vi "test26-MappingRelationshipByLocalRegistration_WithSubcriberName.vi"(8 "error in (no error)":errorcluster, 11 "TestCase in":refnum<class "testcase-CSMBroadcast.lvclass">) -> (0 "error out":errorcluster, 3 "TestCase out":refnum<class "testcase-CSMBroadcast.lvclass">)   [LabVIEW 2017, in "testcase-CSMBroadcast.lvclass"]
uses:
  testcase-CSMBroadcast.lvclass
  caa41fc0-4920-4570-a7eb-0567c3b7bd6c.vi
  <vilib>/addons/_JKI Toolkits/VI Tester/TestCase.llb/TestCase.lvclass
  src/user.lib/_NEVSTOP/Communicable State Machine(CSM)/Communicable State Machine.lvlib
  CSM/CSM-Testcase.lvlib
  C:/Program Files (x86)/National Instruments/LabVIEW 2017/vi.lib/addons/_JKI Toolkits/VI Tester/TestCase.llb/TestCase.lvclass
panel:
  out "Loop Count":i32
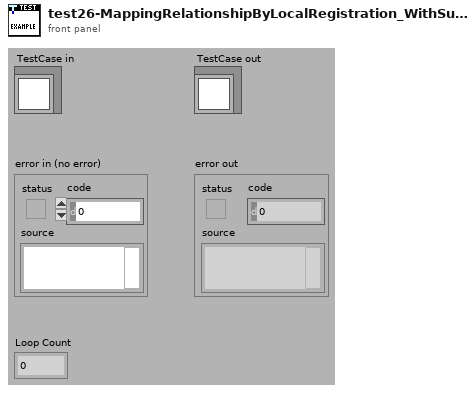
[diagram p1: front panel]
types:
  T1 = cluster{"Status":string, "Source CSM":string, "Target CSM":string, "Target API":string}[]
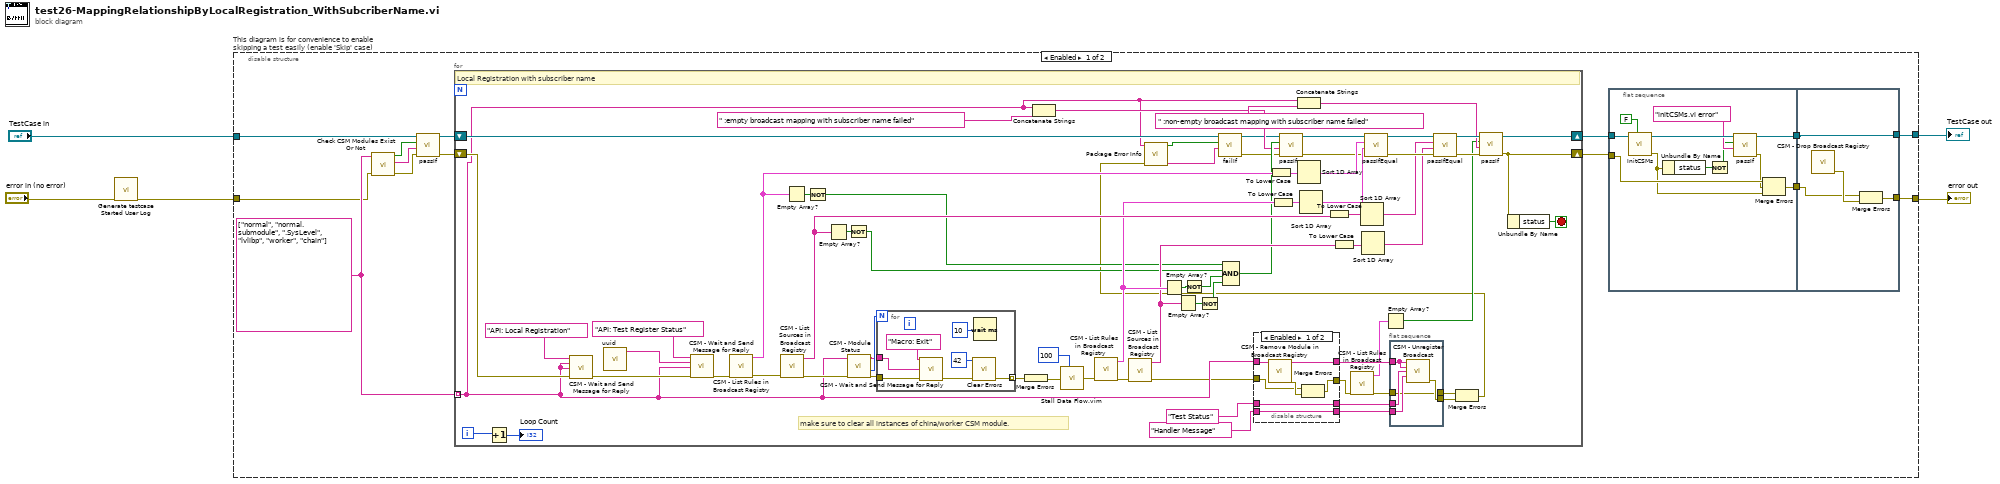
[diagram p0: block diagram]
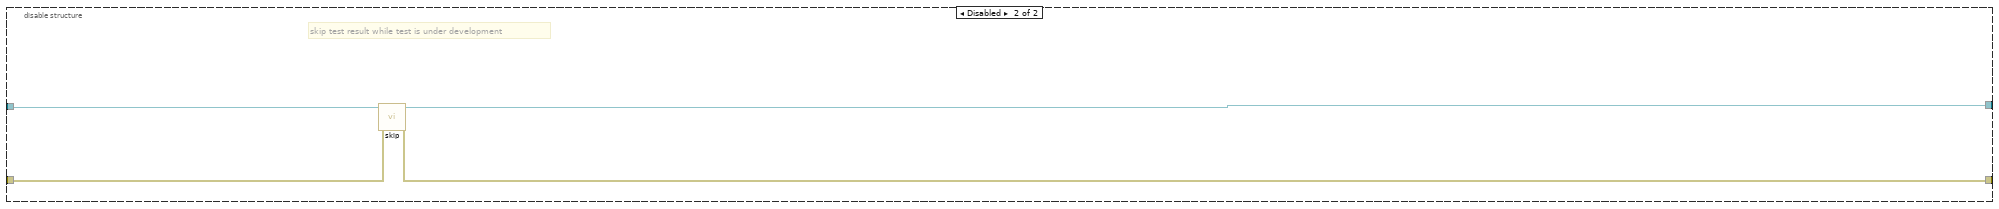
[diagram p3: hidden frame]
diagram:
  n1 = call "Generate testcase Started User Log.vi"("Error In"="error in (no error)") -> ("error out"=w1:errorcluster)  [unwired: 10 in]
  n2 = disable-structure "This diagram is for convenience to enable skipping a test easily (enable 'Skip' case)" shown="Enabled" {
    disable-tunnel: "TestCase in" -> [w15 w132]
    disable-tunnel: [w7 w130] -> w2
    disable-tunnel: [w6 w131] -> w4
    disable-tunnel: w1 -> [w13 w129]
    frame Enabled {
      w16 = string[] ["normal", "normal.submodule", ".SysLevel", "lvlibp", "worker", "chain"]
      n3 = call "Check CSM Modules Exist Or Not.vi"("error in"=w13, "CSM names in"=w16) -> ("error out"=w17:errorcluster, "Debug string"=w18:string, "All Modules Exist?"=w19:bool)  [unwired: 7 in]
      n4 = call-dynamic "passIf.vi"("error in (no error)"=w17, "message (\"\")"=w18, "pass"=w19, "TestCase in"=w15) -> ("error out"=w12:errorcluster, "TestCase out"=w14:refnum<class "testcase-CSMBroadcast.lvclass">)  [unwired: 6 in]
      n5 = for {
        tunnel: w16 -> [w41] mode=indexing
        shift-right: [w71] -> w9
        shift-left: w14 -> [w52]
        shift-right: [w72] -> w8
        shift-left: w12 -> [w62]
        i -> [w86]
        stop <- w99 stop-if-true
        # "make sure to clear all instances of china/worker CSM module."
        # "Local Registration with subscriber name"
        n6 = Increment(x=w86) -> (x+1=→"Loop Count":i32)
        n7 = call "CSM - Wait and Send Message for Reply.vi"("State"="API: Local Registration", "Arguments (\"\")"=w41, "Target Module"=w41, "Error In (No Error)"=w62) -> ("error out"=w104:errorcluster)  [unwired: 8 in, 3 out]
        n8 = call "uuid.vi"() -> ("UUID"=w102:string)  [unwired: 11 in]
        n9 = call "CSM - Wait and Send Message for Reply.vi"("State"="API: Test Register Status", "Arguments (\"\")"=w102, "Target Module"=w41, "Error In (No Error)"=w104) -> ("error out"=w101:errorcluster)  [unwired: 8 in, 3 out]
        n10 = call "CSM - List Rules in Broadcast Registry.vi"("error in (no error)"=w101) -> ("error out"=w98:errorcluster, "Rule Entries"=w84:T1)  [unwired: 8 in, 1 out]
        n11 = call "CSM - List Sources in Broadcast Registry.vi"("error in (no error)"=w98) -> ("error out"=w67:errorcluster, "Broadcast Names"=w81:string[])  [unwired: 9 in]
        n12 = Empty Array?(array=w84) -> (empty?=w83:bool)
        n13 = Not(x=w83) -> (.not. x?=w76:bool)
        n14 = Empty Array?(array=w81) -> (empty?=w82:bool)
        n15 = Not(x=w82) -> (.not. x?=w75:bool)
        n16 = call "CSM - Module Status.vi"("Error In"=w67, "CSM Name"=w41) -> ("error out"=w68:errorcluster, "#Nodes"=w70:i32, "CSM Name (Dup)"=w69:string)  [unwired: 5 in, 2 out]
        n17 = for {
          N: w70 -> [_]
          tunnel: w69 -> [w127]
          tunnel: w68 -> [w126]
          tunnel: [w124] -> w100 mode=indexing
          n18 = call "CSM - Wait and Send Message for Reply.vi"("State"="Macro: Exit", "Target Module"=w127, "Error In (No Error)"=w126) -> ("error out"=w125:errorcluster)  [unwired: 9 in, 3 out]
          n19 = call <vilib>:"Clear Errors.vi"("error in (no error)"=w125, "specific error code to clear (0: all)"=42) -> ("error out"=w124:errorcluster)  [unwired: 4 in, 1 out]
          n20 = Wait (ms)(milliseconds to wait=u32 10) -> ()  [unwired: 1 out]
        }
        n21 = Merge Errors(w100) -> (w56:errorcluster)
        n22 = Concatenate Strings(w41, " :empty broadcast mapping with subscriber name failed" ("string")) -> (w58:string)
        n23 = call "Stall Data Flow.vim"("value in"=w56, "milliseconds to wait"=u32 100) -> ("value out"=w55:errorcluster)  [unwired: 1 out]
        n24 = call "CSM - List Rules in Broadcast Registry.vi"("error in (no error)"=w55) -> ("error out"=w97:errorcluster, "Rule Entries"=w79:T1)  [unwired: 8 in, 1 out]
        n25 = call "CSM - List Sources in Broadcast Registry.vi"("error in (no error)"=w97) -> ("error out"=w40:errorcluster, "Broadcast Names"=w77:string[])  [unwired: 9 in]
        n26 = Empty Array?(array=w79) -> (empty?=w80:bool)
        n27 = Empty Array?(array=w77) -> (empty?=w78:bool)
        n28 = Not(x=w80) -> (.not. x?=w74:bool)
        n29 = Not(x=w78) -> (.not. x?=w73:bool)
        n30 = Compound Arithmetic op=AND(w76, w75, w74, w73) -> (w61:bool)
        n31 = disable-structure shown="Enabled" {
          disable-tunnel: w40 -> [w111 w120]
          disable-tunnel: [w115 w120] -> w47
          disable-tunnel: w41 -> [w116 w121]
          disable-tunnel: "Test Status" ("Status") -> [w113 w119]
          disable-tunnel: "Handler Message" ("Response Message (If \"\", Same as Source Message)") -> [w112 w118]
          disable-tunnel: [w114 w121] -> w48
          disable-tunnel: [w113 w119] -> w46
          disable-tunnel: [w112 w118] -> w45
          frame Enabled {
            n32 = call "CSM - Remove Module in Broadcast Registry.vi"("CSM Name"=w116) -> ("CSM Name (Dup)"=w114:string, "error out"=w117:errorcluster)  [unwired: 13 in]
            n33 = Merge Errors(w111, w117) -> (w115:errorcluster)
          }
          frame Disabled {
          }
        }
        n34 = To Lower Case(string=w84) -> (all lower case string=w96:T1)
        n35 = To Lower Case(string=w79) -> (all lower case string=w95:T1)
        n36 = Concatenate Strings(w41, " :non-empty broadcast mapping with subscriber name failed" ("string")) -> (w57:string)
        n37 = Sort 1D Array(array=w96) -> (sorted array=w94:T1)
        n38 = Sort 1D Array(array=w95) -> (sorted array=w93:T1)
        n39 = To Lower Case(string=w81) -> (all lower case string=w90:string[])
        n40 = To Lower Case(string=w77) -> (all lower case string=w89:string[])
        n41 = call "CSM - List Rules in Broadcast Registry.vi"("error in (no error)"=w47) -> ("error out"=w43:errorcluster, "Rule Entries"=w37:T1)  [unwired: 8 in, 1 out]
        n42 = Sort 1D Array(array=w90) -> (sorted array=w88:string[])
        n43 = Sort 1D Array(array=w89) -> (sorted array=w87:string[])
        n44 = Empty Array?(array=w37) -> (empty?=w36:bool)
        n45 = flat-sequence {
          tunnel: w48 -> [w110]
          tunnel: w46 -> [w109]
          tunnel: w45 -> [w108]
          tunnel: [w107] -> w44
          tunnel: w43 -> [w106]
          tunnel: [w106] -> w42
          frame #0 {
            n46 = call "CSM - Unregister Broadcast.vi"("CSM Name(Empty for Broadcast Event)"=w110, "Source CSM Name (* as Default)"=w110, "Trigger"=w109, "API (\"*\" as Default)"=w108) -> ("error out"=w107:errorcluster)  [unwired: 10 in, 1 out]
          }
        }
        n47 = Merge Errors(w42, w44) -> (w35:errorcluster)
        n48 = call "Package Error Info.vi"("error in"=w35, "String in"=w41) -> ("packed error info out"=w49:string, "error status"=w50:bool)  [unwired: 8 in]
        n49 = call-dynamic "failIf.vi"("message (\"\")"=w49, "fail"=w50, "TestCase in"=w52) -> ("error out"=w51:errorcluster, "TestCase out"=w53:refnum<class "testcase-CSMBroadcast.lvclass">)  [unwired: 7 in]
        n50 = call-dynamic "passIf.vi"("error in (no error)"=w51, "message (\"\")"=w58, "pass"=w61, "TestCase in"=w53) -> ("error out"=w63:errorcluster, "TestCase out"=w64:refnum<class "testcase-CSMBroadcast.lvclass">)  [unwired: 6 in]
        n51 = call-dynamic "passIfEqual.vi"("error in (no error)"=w63, "y"=w93, "x"=w94, "TestCase in"=w64) -> ("error out"=w91:errorcluster, "TestCase out"=w92:refnum<class "testcase-CSMBroadcast.lvclass">)  [unwired: 6 in]
        n52 = call-dynamic "passIfEqual.vi"("error in (no error)"=w91, "y"=w87, "x"=w88, "TestCase in"=w92) -> ("error out"=w65:errorcluster, "TestCase out"=w66:refnum<class "testcase-CSMBroadcast.lvclass">)  [unwired: 6 in]
        n53 = call-dynamic "passIf.vi"("error in (no error)"=w65, "message (\"\")"=w57, "pass"=w36, "TestCase in"=w66) -> ("error out"=w72:errorcluster, "TestCase out"=w71:refnum<class "testcase-CSMBroadcast.lvclass">)  [unwired: 6 in]
        n54 = Unbundle By Name(w72) -> ("status"=w99:bool)
      }
      n55 = flat-sequence {
        tunnel: w9 -> [w30]
        tunnel: [w27] -> w11
        tunnel: w8 -> [w24]
        tunnel: [w21] -> w10
        tunnel: w11 -> [w33]
        tunnel: [w33] -> w7
        tunnel: [w32] -> w6
        tunnel: w10 -> [w31]
        frame #0 {
          n56 = call "InitCSMs.vi"("Enable building lvlibp?"=FALSE, "testcase-CSMStatus in"=w30) -> ("error out"=w22:errorcluster, "testcase-CSMStatus out"=w28:refnum<class "testcase-CSMBroadcast.lvclass">)  [unwired: 8 in]
          n57 = Unbundle By Name(w22) -> ("status"=w26:bool)
          n58 = Not(x=w26) -> (.not. x?=w20:bool)
          n59 = call-dynamic "passIf.vi"("message (\"\")"="initCSMs.vi error" ("message (\"\")"), "pass"=w20, "TestCase in"=w28) -> ("error out"=w23:errorcluster, "TestCase out"=w27:refnum<class "testcase-CSMBroadcast.lvclass">)  [unwired: 7 in]
          n60 = Merge Errors(w24, w23, w22) -> (w21:errorcluster)
        }
        frame #1 {
          n61 = call "CSM - Drop Broadcast Registry.vi"() -> ("error out"=w34:errorcluster)  [unwired: 15 in]
          n62 = Merge Errors(w31, w34) -> (w32:errorcluster)
        }
      }
    }
    frame Disabled {
      # "skip test result while test is under development"
      n63 = call <vilib>:"skip.vi"("error in (no error)"=w129, "TestCase in"=w132) -> ("error out"=w131:errorcluster, "TestCase out"=w130:refnum<class "testcase-CSMBroadcast.lvclass">)  [unwired: 8 in]
    }
  }
  "error out" <- w4
  "TestCase out" <- w2
